vi "Initialise Base Actor.vi"(6 "Name":string, 7 "Tick Period [100 ms]":dbl=0.1, 8 "error in (no error)":errorcluster, 10 "Received Messages Channel":refnum<user-event>, 11 "Actor in":refnum<class "Actor.lvclass">) -> (0 "error out":errorcluster, 3 "Actor out":refnum<class "Actor.lvclass">)   [LabVIEW 2020, in "Actor.lvclass"]
uses:
  Actor.lvclass
  Sequencer/Sequencer.lvclass
  Message.ctl
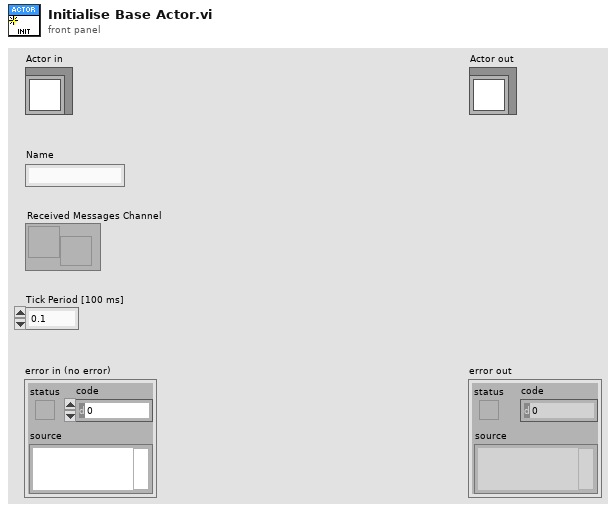
[diagram p1: front panel]
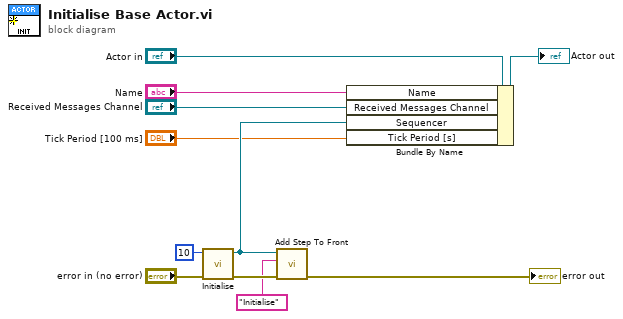
[diagram p0: block diagram]
diagram:
  n1 = call "Initialise.vi"("error in (no error)"="error in (no error)", "Max Steps (10)"=10) -> ("error out"=w5:errorcluster, "Sequencer out"=w3:refnum<class "Sequencer.lvclass">)  [unwired: 8 in]
  n2 = call "Add Step To Front.vi"("error in (no error)"=w5, "Step Name"="Initialise", "Sequencer in"=w3) -> ("error out"=→"error out":errorcluster)  [unwired: 8 in]
  n3 = Bundle By Name(cluster="Actor in", "Name"="Name", "Received Messages Channel"="Received Messages Channel", "Sequencer"=w3, "Tick Period [s]"="Tick Period [100 ms]") -> (→"Actor out":refnum<class "Actor.lvclass">)
